vi "ReadAOs.vi"(3 "error in":errorcluster, 4 "substring (\"\")":string="Dev3/_", 5 "array":cluster{dbl, string, "Output Channels":tag}[](array[cluster])) -> (0 "error out 2":errorcluster, 1 "AO1":dbl, 2 "AO0":dbl)   [LabVIEW 2013]
uses:
  <vilib>/DAQmx/read.llb/DAQmx Read (Analog 1D DBL NChan 1Samp).vi
  <vilib>/DAQmx/create/channels.llb/DAQmx Create Channel (AI-Voltage-Basic).vi
  <vilib>/DAQmx/miscellaneous.llb/DAQmx Fill In Error Info.vi
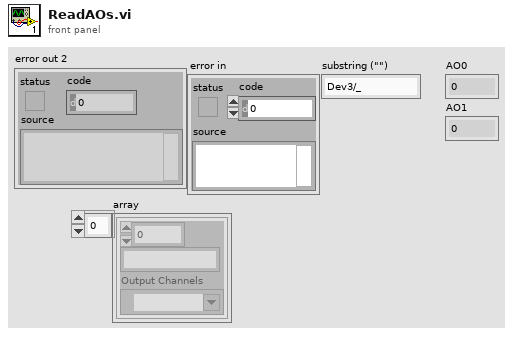
[diagram p1: front panel]
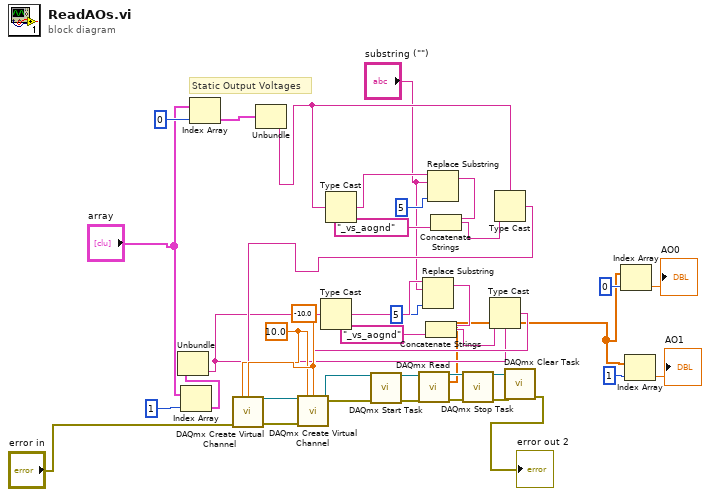
[diagram p0: block diagram]
diagram:
  w35 = -10.0 ("minimum value")
  w34 = 10.0 ("maximum value")
  # "Static Output Voltages"
  n1 = Index Array(array="array", index=1) -> (element=w10:cluster{dbl, string, "Output Channels":tag})
  n2 = Unbundle(w10) -> ("Output Channels"=w20:tag)  [unwired: 2 out]
  n3 = Index Array(array="array", index=0) -> (element=w9:cluster{dbl, string, "Output Channels":tag})
  n4 = Unbundle(w9) -> ("Output Channels"=w26:tag)  [unwired: 2 out]
  n5 = Type Cast(x=w20) -> (*(type *) &x=w17:string)  [unwired: 1 in]
  n6 = Type Cast(x=w26) -> (*(type *) &x=w21:string)  [unwired: 1 in]
  n7 = Replace Substring(2:5 ("length (len. of substring)"), 4:"substring (\"\")", 5:w17) -> (1:w15:string)  [unwired: 1 in, 1 out]
  n8 = Concatenate Strings(w15, "_vs_aognd" ("string")) -> (w13:string)
  n9 = Replace Substring(2:5 ("length (len. of substring)"), 4:"substring (\"\")", 5:w21) -> (1:w23:string)  [unwired: 1 in, 1 out]
  n10 = Concatenate Strings(w23, "_vs_aognd" ("string")) -> (w25:string)
  n11 = Type Cast(type=w20, x=w13) -> (*(type *) &x=w29:tag)
  n12 = Type Cast(type=w26, x=w25) -> (*(type *) &x=w27:tag)
  n13 = call-poly <vilib>:"DAQmx Create Virtual Channel.vi"("maximum value"=w34, "minimum value"=w35, "physical channels"=w27, "error in"="error in") -> ("task out"=w28:refnum<k21>, "error out"=w33:errorcluster)  [unwired: 10 in]
  n14 = call-poly <vilib>:"DAQmx Create Virtual Channel.vi"("task in"=w28, "maximum value"=w34, "minimum value"=w35, "physical channels"=w29, "error in"=w33) -> ("task out"=w38:refnum<k21>, "error out"=w39:errorcluster)  [unwired: 9 in]
  n15 = call <vilib>:"DAQmx Start Task.vi"("task/channels in"=w38, "error in"=w39) -> ("task out"=w36:refnum<k21>, "error out"=w37:errorcluster)  [unwired: 12 in]
  n16 = call-poly <vilib>:"DAQmx Read.vi"("task/channels in"=w36, "error in"=w37) -> ("task out"=w19:refnum<k21>, "data"=w6:dbl[], "error out"=w32:errorcluster)  [unwired: 11 in]
  n17 = call <vilib>:"DAQmx Stop Task.vi"("task/channels in"=w19, "error in"=w32) -> ("task out"=w18:refnum<k21>, "error out"=w31:errorcluster)  [unwired: 12 in]
  n18 = call <vilib>:"DAQmx Clear Task.vi"("task in"=w18, "error in"=w31) -> ("error out"=→"error out 2":errorcluster)  [unwired: 13 in]
  n19 = Index Array(array=w6, index=0) -> (element=→"AO0":dbl)
  n20 = Index Array(array=w6, index=1) -> (element=→"AO1":dbl)
